vi "ReadBundler.vi"(2 "reference":refnum<vi>) -> (1 "Bundler":T6)   [LabVIEW 2013]
uses:
  <vilib>/Utility/miscctls.llb/LVBoundsTypeDef.ctl
  <vilib>/Utility/miscctls.llb/LVRectTypeDef.ctl
  <vilib>/Utility/miscctls.llb/LVPositionTypeDef.ctl
  <vilib>/Utility/miscctls.llb/LVBreakpointStatusEnum.ctl
  <vilib>/picture/picture.llb/imagedata.ctl
panel:
  out "error out":errorcluster
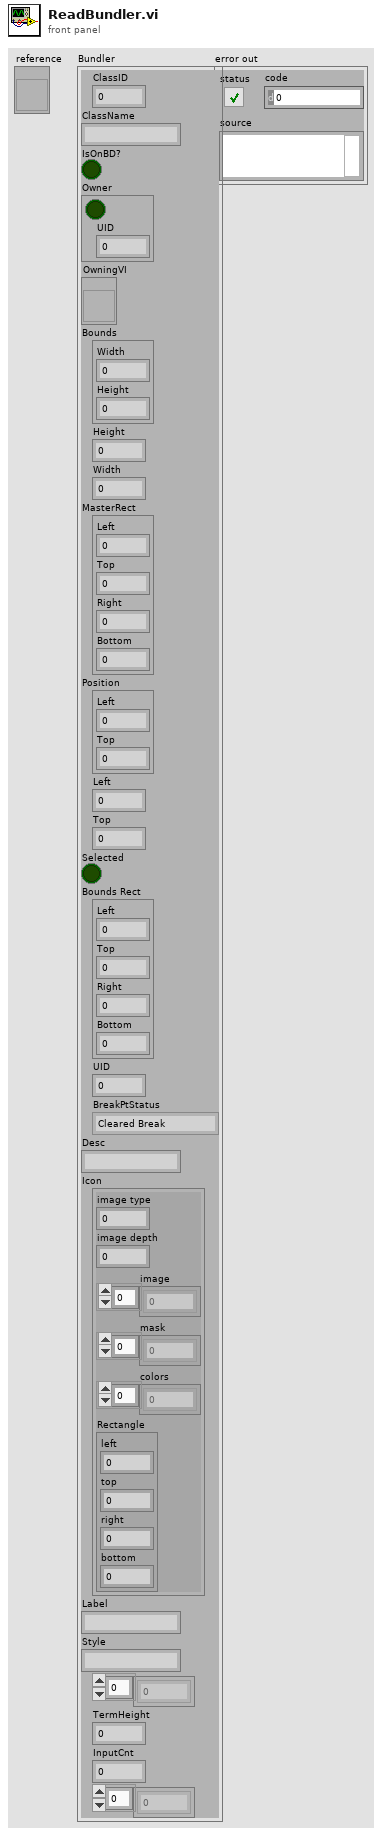
[diagram p1: front panel]
types:
  T1 = typedef "LVBoundsTypeDef.ctl" = cluster{"Width":u32, "Height":u32}
  T2 = typedef "LVRectTypeDef.ctl" = cluster{"Left":i16, "Top":i16, "Right":i16, "Bottom":i16}
  T3 = typedef "LVPositionTypeDef.ctl" = cluster{"Left":i32, "Top":i32}
  T4 = typedef "LVBreakpointStatusEnum.ctl" = enum8{"Cleared Break", "Enabled Break", "Disabled Break"}
  T5 = typedef "imagedata.ctl" = cluster{"image type":i32, "image depth":i32, "image":u8[], "mask":u8[], "colors":u32[], "Rectangle":cluster{"left":i16, "top":i16, "right":i16, "bottom":i16}}
  T6 = cluster{"ClassID":u32, "ClassName":string, "IsOnBD?":bool, "Owner":cluster{bool, "UID":i32}, "OwningVI":refnum<vi>, "Bounds":T1, "Height":u32, "Width":u32, "MasterRect":T2, "Position":T3, "Left":i32, "Top":i32, "Selected":bool, "Bounds Rect":T2, "UID":i32, "BreakPtStatus":T4, "Desc":string, "Icon":T5, "Label":string, "Style":string, "Terms[]":i32[], "TermHeight":i32, "InputCnt":i32, "InputTerms[]":i32[]}
  T7 = cluster{"ClassID":u32, "ClassName":string, "IsOnBD?":bool, "Cluster":cluster{bool, "UID":i32}, "OwningVI":refnum<vi>, "Bounds":T1, "Height":u32, "Width":u32, "MasterRect":T2, "Position":T3, "Left":i32, "Top":i32, "Selected":bool, "Bounds Rect":T2, "UID":i32, "BreakPtStatus":T4, "Desc":string, "Icon":T5, "Text":string, "Style":string, i32[], "TermHeight":i32, "InputCnt":i32, i32[]}
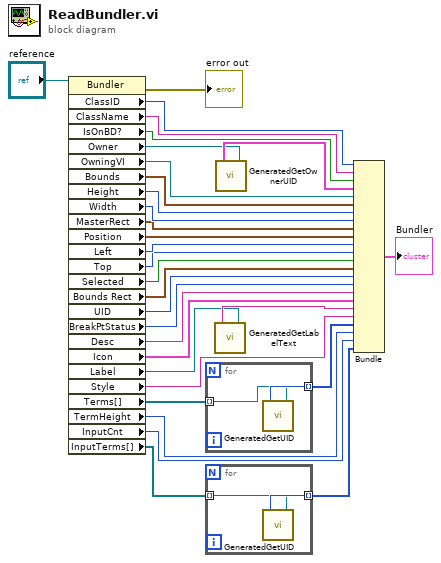
[diagram p0: block diagram]
diagram:
  n1 = property class="Bundler"(reference="reference") -> (error out=→"error out":errorcluster, "ClassID"=w30:u32, "ClassName"=w29:string, "IsOnBD?"=w28:bool, "Owner"=w26:refnum<vi>, "OwningVI"=w25:refnum<vi>, "Bounds"=w24:T1, "Height"=w23:u32, "Width"=w22:u32, "MasterRect"=w21:T2, "Position"=w20:T3, "Left"=w19:i32, "Top"=w18:i32, "Selected"=w17:bool, "Bounds Rect"=w16:T2, "UID"=w15:i32, "BreakPtStatus"=w14:T4, "Desc"=w13:string, "Icon"=w12:T5, "Label"=w10:refnum<vi>, "Style"=w9:string, "Terms[]"=w7:refnum<vi>[], "TermHeight"=w6:i32, "InputCnt"=w5:i32, "InputTerms[]"=w3:refnum<vi>[])  [unwired: 1 in, 1 out]
  n2 = for {
    tunnel: [w33] -> w8 mode=indexing
    tunnel: w7 -> [w32] mode=indexing
    n3 = call "GeneratedGetUID.vi"("Text in"=w32) -> ("UID"=w33:i32)
  }
  n4 = for {
    tunnel: [w35] -> w4 mode=indexing
    tunnel: w3 -> [w34] mode=indexing
    n5 = call "GeneratedGetUID.vi"("Text in"=w34) -> ("UID"=w35:i32)
  }
  n6 = call "GeneratedGetLabelText.vi"("Text in"=w10) -> ("Text"=w11:string)
  n7 = call "GeneratedGetOwnerUID.vi"("Generic in"=w26) -> ("Cluster"=w27:cluster{bool, "UID":i32})
  n8 = Bundle("ClassID"=w30, "ClassName"=w29, "IsOnBD?"=w28, "Cluster"=w27, "OwningVI"=w25, "Bounds"=w24, "Height"=w23, "Width"=w22, "MasterRect"=w21, "Position"=w20, "Left"=w19, "Top"=w18, "Selected"=w17, "Bounds Rect"=w16, "UID"=w15, "BreakPtStatus"=w14, "Desc"=w13, "Icon"=w12, "Text"=w11, "Style"=w9, w8, "TermHeight"=w6, "InputCnt"=w5, w4) -> (→"Bundler":T7)  [unwired: 1 in]
